vi "Simple Stream.vi"() -> ()   [LabVIEW 2016, in "Lab Streaming Layer.lvlib"]
uses:
  Lab Streaming Layer.lvlib
  Custom Controls/lsl_channel_format.ctl
panel:
  out "Array":dbl[][](array[numeric])
  out "Have Consumers":i32
  out "function return":i32
  in  "stop":bool
  out "source id":string
  out "nominal samplerate":dbl
  out "name":string
  out "channel bytes":i32
  out "channel count":i32
  out "xml":string
  out "version":i32
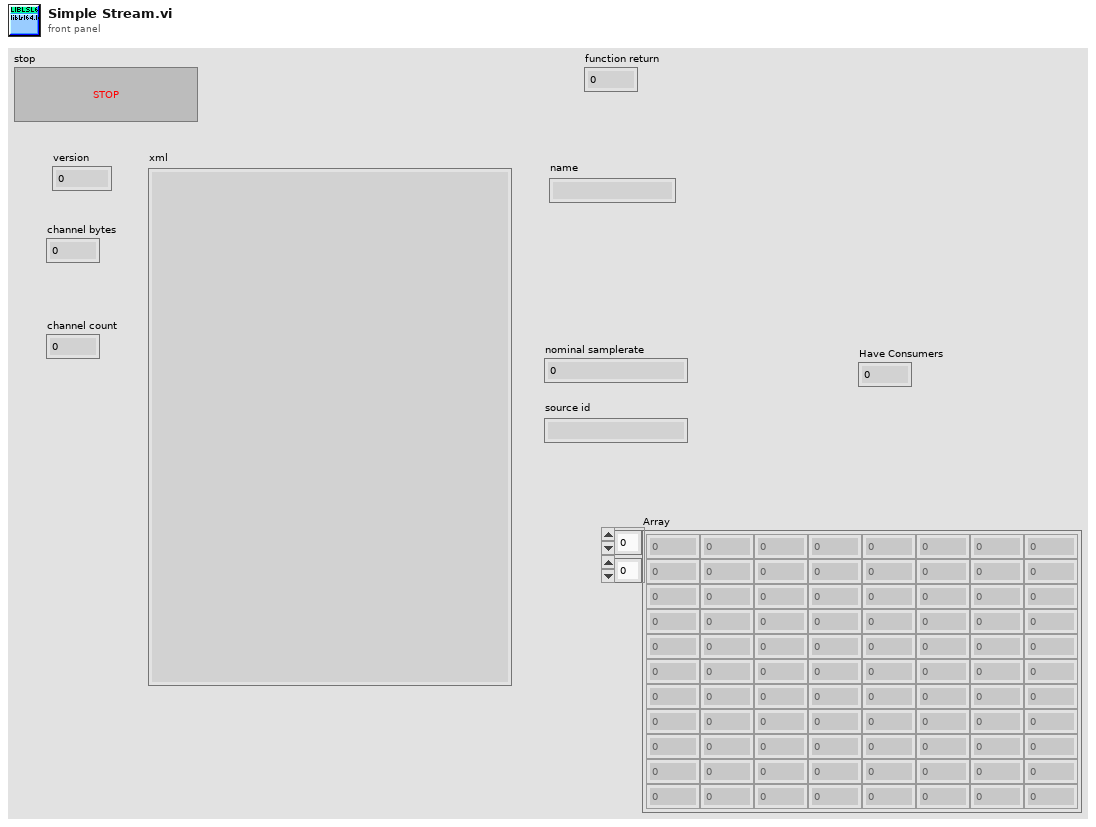
[diagram p1: front panel]
types:
  T1 = typedef "Lab Streaming Layer.lvlib/lsl_channel_format.ctl" = u32
  T2 = typedef "Lab Streaming Layer.lvlib/lsl_streaminfo.ctl" = u64
  T3 = typedef "Lab Streaming Layer.lvlib/lsl_outlet.ctl" = u64
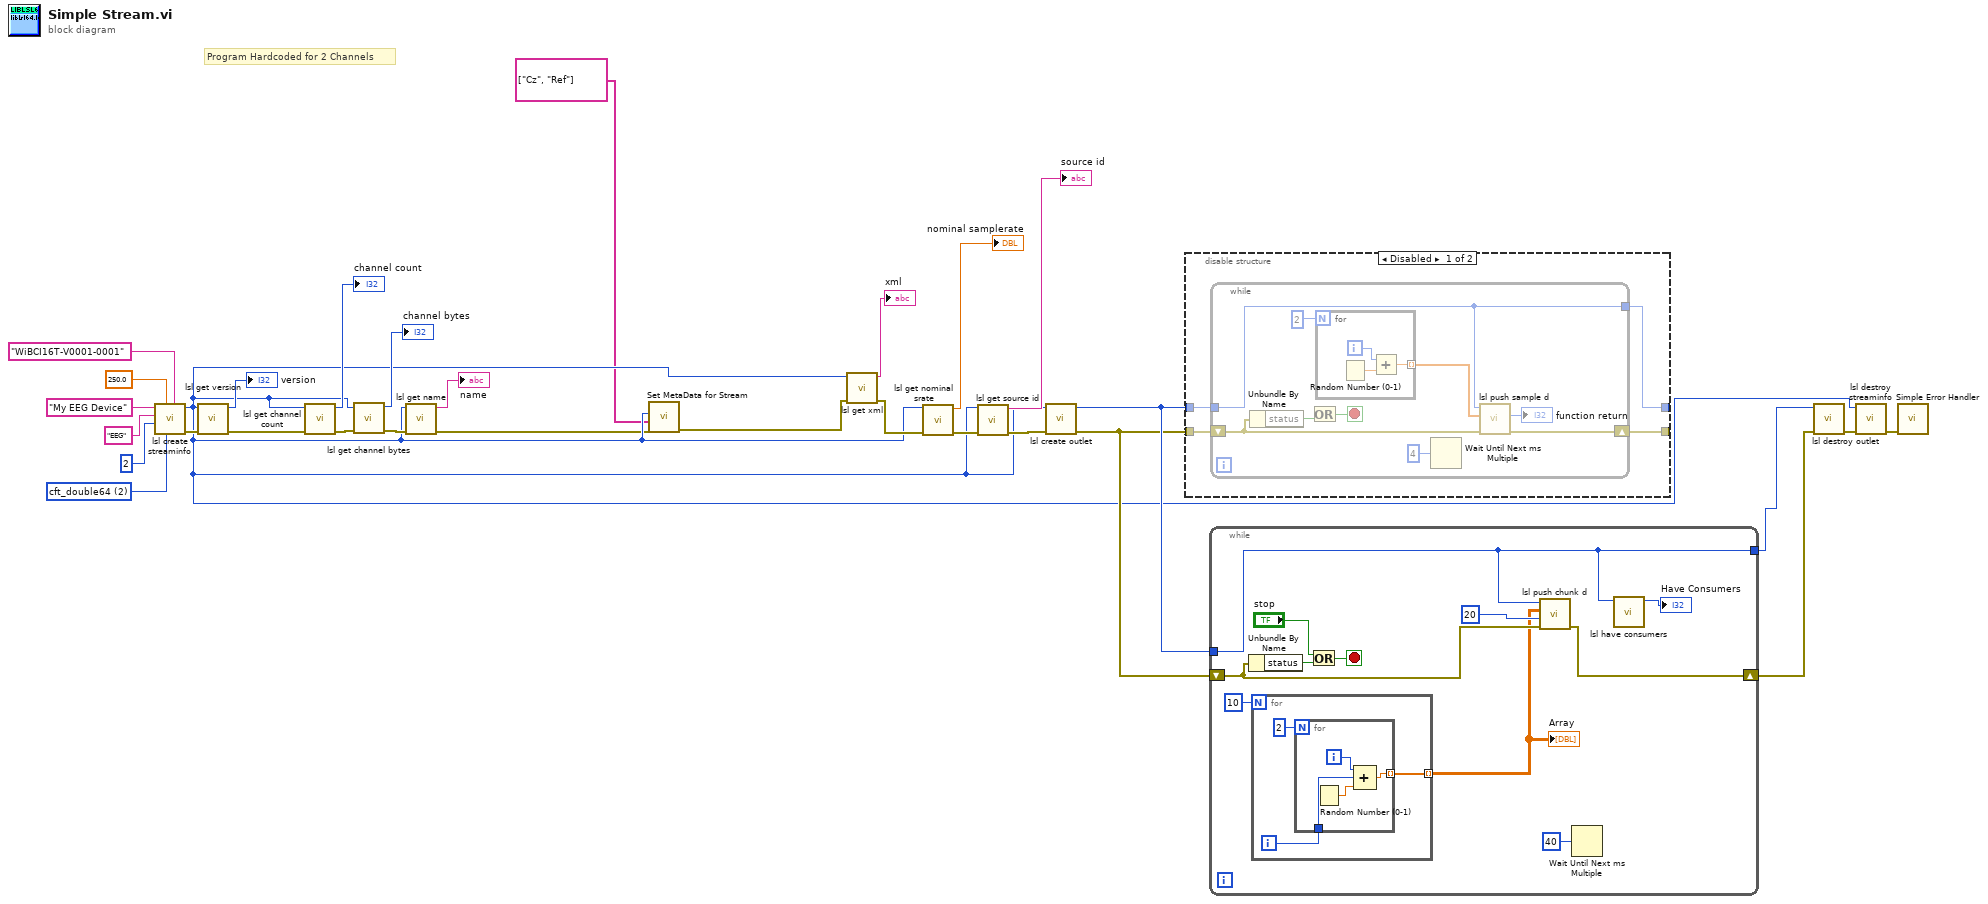
[diagram p0: block diagram]
diagram:
  w25 = T1 2 items=["cft_float32"=1, "cft_double64"=2, "cft_string"=3, "cft_int32"=4, "cft_int16"=5, "cft_int8"=6, "cft_int64"=7, "cft_undefined"=0] ("channel_format")
  # "Program Hardcoded for 2 Channels"
  n1 = call "lsl create streaminfo.vi"("source_id"="WiBCI16T-V0001-0001", "channel_format"=w25, "samplingrate"=250.0, "channel_count"=2, "type"="EEG", "name"="My EEG Device") -> ("error out"=w24:errorcluster, "streaminfo"=w4:T2)  [unwired: 4 in]
  n2 = call "lsl get version.vi"("error in"=w24, "streaminfo"=w4) -> ("error out"=w7:errorcluster, "version"=→"version":i32)  [unwired: 8 in]
  n3 = call "lsl get channel count.vi"("error in (no error)"=w7, "streaminfo"=w4) -> ("error out"=w21:errorcluster, "channel count"=→"channel count":i32)  [unwired: 8 in]
  n4 = call "lsl get channel bytes.vi"("error in (no error)"=w21, "streaminfo"=w4) -> ("error out"=w19:errorcluster, "channel bytes"=→"channel bytes":i32)  [unwired: 8 in]
  n5 = call "lsl get name.vi"("error in (no error)"=w19, "streaminfo"=w4) -> ("error out"=w2:errorcluster, "name"=→"name":string)  [unwired: 8 in]
  n6 = call "Set MetaData for Stream.vi"("error in"=w2, "Ch Names"=string[] ["Cz", "Ref"], "streaminfo"=w4) -> ("error out"=w1:errorcluster)  [unwired: 8 in]
  n7 = call "lsl get xml.vi"("error in (no error)"=w1, "streaminfo"=w4) -> ("error out"=w5:errorcluster, "xml"=→"xml":string)  [unwired: 8 in]
  n8 = call "lsl get nominal srate.vi"("error in (no error)"=w5, "streaminfo"=w4) -> ("error out"=w16:errorcluster, "nominal samplerate"=→"nominal samplerate":dbl)  [unwired: 8 in]
  n9 = call "lsl get source id.vi"("error in (no error)"=w16, "streaminfo"=w4) -> ("error out"=w14:errorcluster, "source id"=→"source id":string)  [unwired: 8 in]
  n10 = call "lsl create outlet.vi"("error in (no error)"=w14, "streaminfo"=w4) -> ("error out"=w10:errorcluster, "outlet"=w11:T3)  [unwired: 8 in]
  n11 = disable-structure shown="Disabled" {
    disable-tunnel: w11 -> [w34 _]
    disable-tunnel: w10 -> [w33 _]
    disable-tunnel: [w32 _] -> _
    disable-tunnel: [w31 _] -> _
    frame Disabled {
      n12 = while {
        tunnel: w34 -> [w35]
        shift-right: [w39] -> w31
        shift-left: w33 -> [w40]
        tunnel: [w35] -> w32
        stop <- w41 stop-if-true
        n13 = Unbundle By Name(w40) -> ("status"=w42:bool)
        n14 = Or(y=w42) -> (x .or. y?=w41:bool)  [unwired: 1 in]
        n15 = for {
          N: 2 -> [_]
          tunnel: [w45] -> w38 mode=indexing
          i -> [w44]
          n16 = Random Number (0-1)() -> (number: 0 to 1=w46:dbl)
          n17 = Add(x=w44, y=w46) -> (x+y=w45:dbl)
        }
        n18 = Wait Until Next ms Multiple(millisecond multiple=u32 4) -> ()  [unwired: 1 out]
        n19 = call "lsl push sample d.vi"("error in (no error)"=w40, "data"=w38, "outlet"=w35) -> ("error out"=w39:errorcluster, "function return"=→"function return":i32)  [unwired: 7 in]
      }
    }
    frame Enabled {
    }
  }
  n20 = while {
    tunnel: w11 -> [w48]
    shift-right: [w53] -> w8
    shift-left: w10 -> [w54]
    tunnel: [w48] -> w9
    stop <- w56 stop-if-true
    n21 = Unbundle By Name(w54) -> ("status"=w57:bool)
    n22 = for {
      N: 10 -> [_]
      tunnel: [w59] -> w49 mode=indexing
      i -> [w58]
      n23 = for {
        N: 2 -> [_]
        tunnel: [w64] -> w59 mode=indexing
        tunnel: w58 -> [w62]
        i -> [w63]
        n24 = Random Number (0-1)() -> (number: 0 to 1=w61:dbl)
        n25 = Compound Arithmetic op=ADD(w63, w62, w61) -> (w64:dbl)
      }
    }
    "Array" <- w49
    n26 = Or(x="stop", y=w57) -> (x .or. y?=w56:bool)
    n27 = call "lsl push chunk d.vi"("error in (no error)"=w54, "data_elements"=i64 20, "data"=w49, "outlet"=w48) -> ("error out"=w53:errorcluster)  [unwired: 6 in, 1 out]
    n28 = Wait Until Next ms Multiple(millisecond multiple=u32 40) -> ()  [unwired: 1 out]
    n29 = call "lsl have consumers.vi"("outlet"=w48) -> ("Have Consumers"=→"Have Consumers":i32)  [unwired: 9 in, 1 out]
  }
  n30 = call "lsl destroy outlet.vi"("error in (no error)"=w8, "outlet"=w9) -> ("error out"=w12:errorcluster)  [unwired: 9 in]
  n31 = call "lsl destroy streaminfo.vi"("error in (no error)"=w12, "streaminfo"=w4) -> ("error out"=w13:errorcluster)  [unwired: 9 in]
  n32 = call <vilib>:"Simple Error Handler.vi"("error in (no error)"=w13) -> ()  [unwired: 4 in, 5 out]
